vi "ComplexWaveformVisualizer.vi"(6 "new?":bool=TRUE, 8 "imag":dbl[](array[numeric]), 9 "real":dbl[](array[numeric]), 10 "dt":dbl format="%#_13g", 11 "t0":dbl format="%#_13g") -> (0 "error out":errorcluster)   [LabVIEW 2018, in "lvnetviz.lvlib" / "ComplexWaveform.lvclass"]
uses:
  ComplexWaveform.lvclass
  37a200e1-ebed-4a42-aca9-62fa0edddda8.vi
  563f4c1e-5713-48a9-8981-6f50fa41d22c.vi
  e92ec0bc-6cb3-4747-b161-0f80a961e92f.vi
  60cc32db-fe2c-4d93-b9a7-8d3187e357da.vi
  692aab13-ca21-4d55-90b4-8dcecc026462.vi
  02b4f178-3a94-4fae-b2df-360b2a148257.vi
  3b6274d3-9685-4d49-9d46-acf0fd8be449.vi
  563f4c1e-5713-48a9-8981-6f50fa41d22c.vi/40b995cc-7a2b-45c3-8b81-c77e08a5a566.vi
  e92ec0bc-6cb3-4747-b161-0f80a961e92f.vi/273ea279-4d78-4cbc-b357-74e972452477.vi
  <vilib>/Analysis/2dsp.llb/Unwrap Phase.vi
  <vilib>/Analysis/2dsp.llb/FFT.vi
  <vilib>/Analysis/2dsp.llb/Complex FFT.vi
  e92ec0bc-6cb3-4747-b161-0f80a961e92f.vi/273ea279-4d78-4cbc-b357-74e972452477.vi/7830e0d0-7296-4e8f-a228-935442eb8294.vi
  <vilib>/Utility/error.llb/Error Cluster From Error Code.vi
panel:
  in  "Tab Control":enum32{"Traces", "Statistics"}(tab)
  out "Waveform Graph":cluster{"t0":dbl, "dt":dbl, "real":dbl[]}[](graph)
  in  "Plot Type":T1(ring)=enum."Power vs. Frequency"
  out "Table Control":string[][](table)
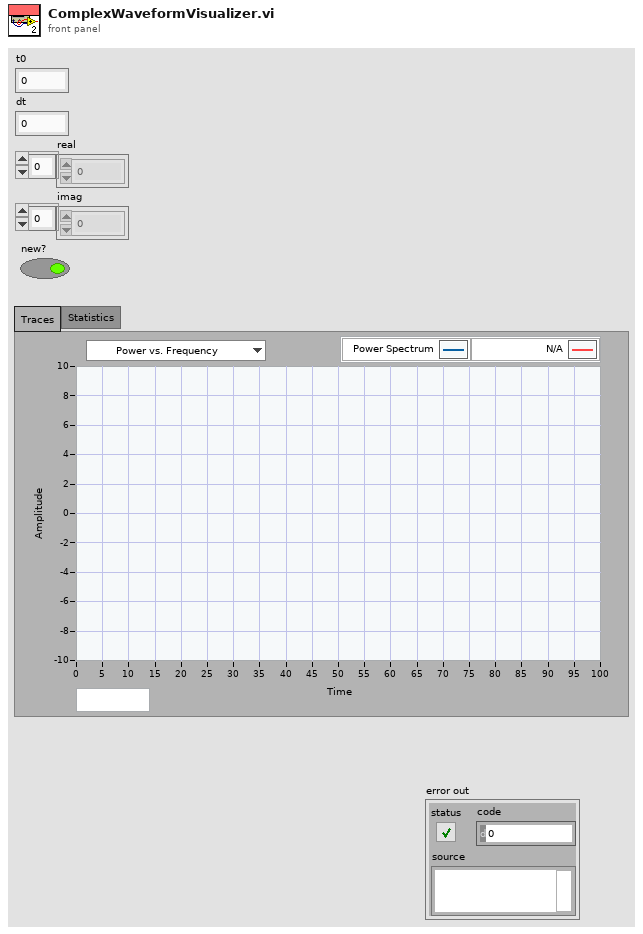
[diagram p1: front panel]
types:
  T1 = enum16{"IQ vs. Time", "Power vs. Time", "Phase vs. Time", "Unwrapped Phase vs. Time", "Delta Phase vs. Time", "Frequency vs. Time", "Power vs. Frequency", "Phase vs. Frequency"}
  T2 = cluster{"t0":dbl, "dt":dbl, "Unwrapped Phase":dbl[]}
  T3 = cluster{"t0":dbl, "dt":dbl, "Unwrapped Phase":dbl[]}[]
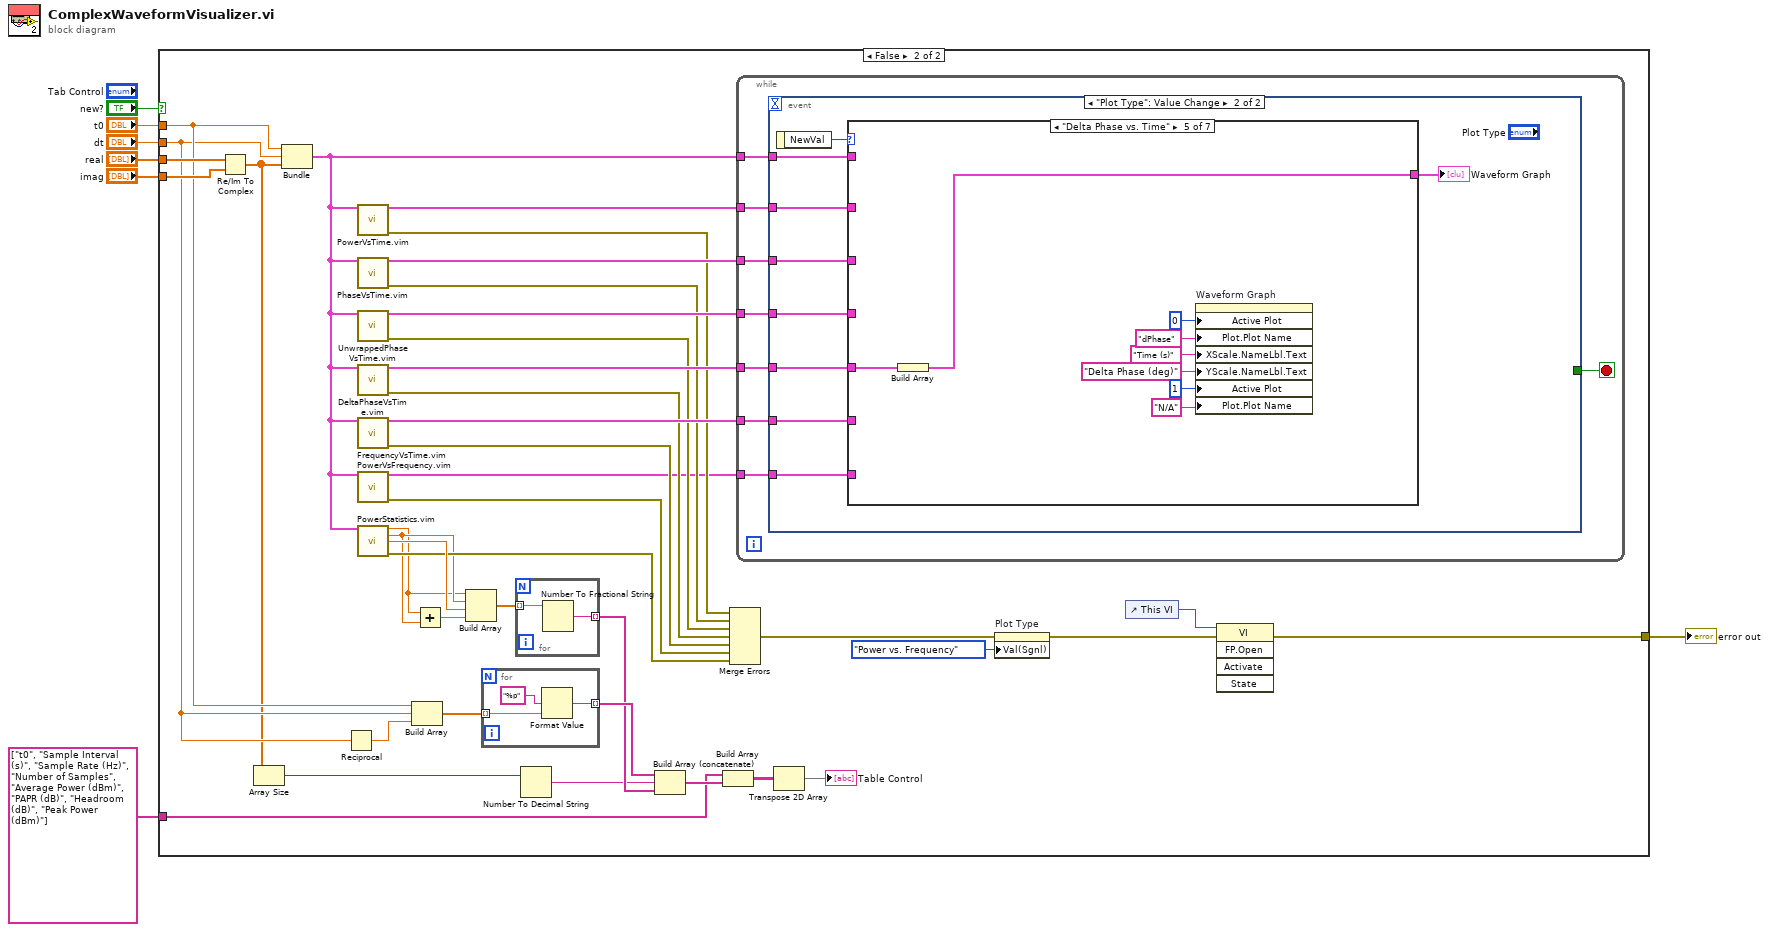
[diagram p0: block diagram]
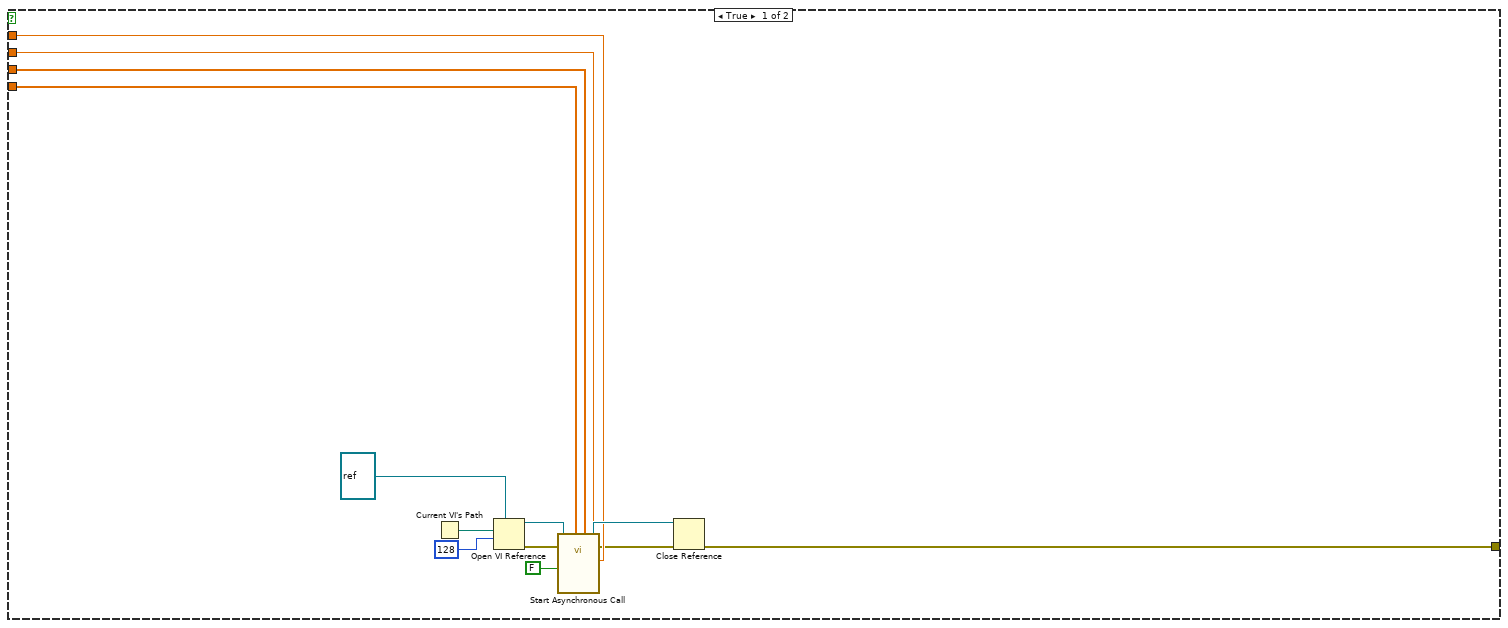
[diagram p2: hidden frame]
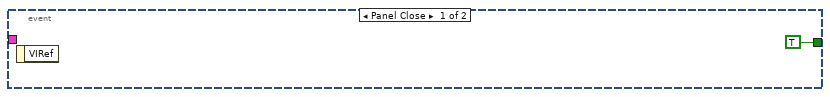
[diagram p3: hidden frame]
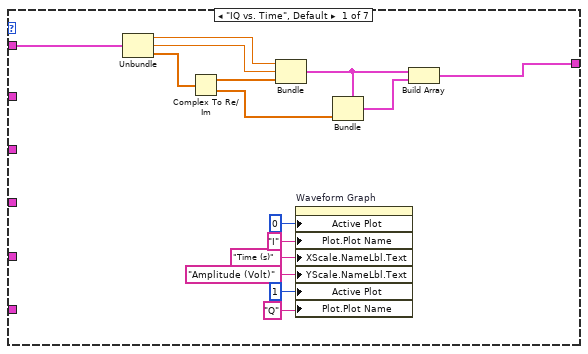
[diagram p4: hidden frame]
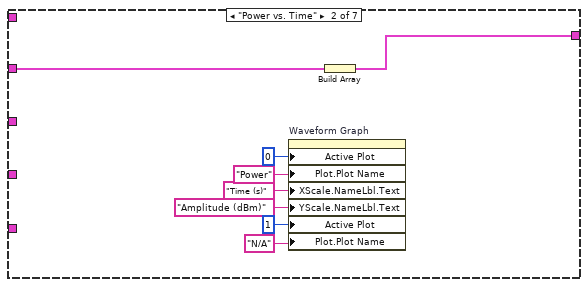
[diagram p5: hidden frame]
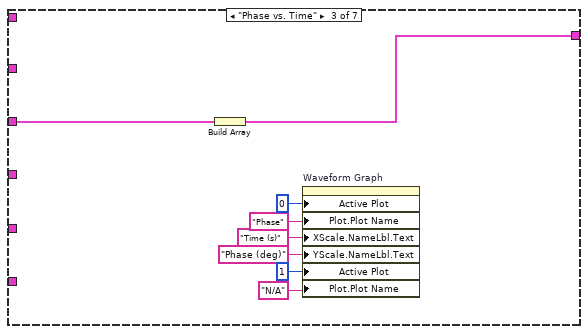
[diagram p6: hidden frame]
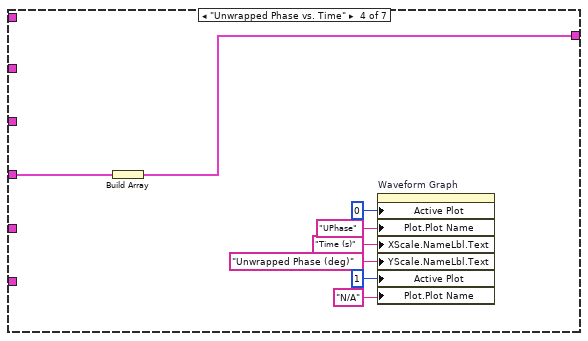
[diagram p7: hidden frame]
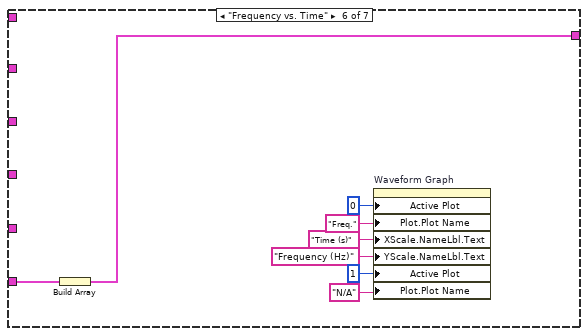
[diagram p8: hidden frame]
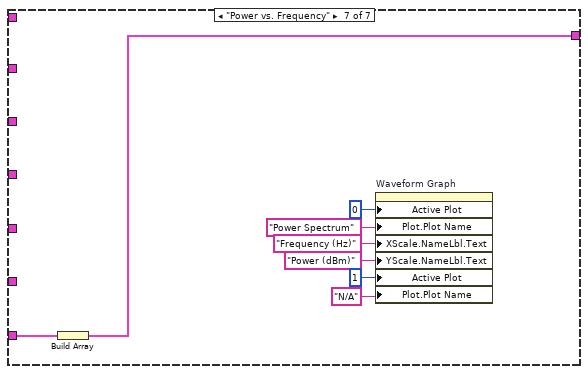
[diagram p9: hidden frame]
diagram:
  n1 = case shown="False" "new?" {
    tunnel: "imag" -> [w12 w52]
    tunnel: "real" -> [w13 w53]
    tunnel: "t0" -> [w15 w48]
    tunnel: "dt" -> [w14 w41]
    tunnel: [w9 w58] -> w2
    tunnel: string[] ["t0", "Sample Interval (s)", "Sample Rate (Hz)", "Number of Samples", "Average Power (dBm)", "PAPR (dB)", "Headroom (dB)", "Peak Power (dBm)"] -> [_ w35]
    frame True {
      n2 = Current VI's Path() -> (path=w20:path)
      n3 = Open VI Reference(type specifier VI Refnum (for type only)=refnum<vi> refnum, vi path=w20, options=128) -> (vi reference=w17:refnum<vi>, error out=w11:errorcluster)  [unwired: 3 in]
      n4 = call-by-ref "Start Asynchronous Call"(reference=w17, error in=w11, "Create New?"=FALSE, "imag"=w12, "real"=w13, "dt"=w14, "t0"=w15) -> (reference out=w16:refnum<vi>, error out=w10:errorcluster)  [unwired: 6 in, 1 out]
      n5 = Close Reference(reference=w16, error in (no error)=w10) -> (error out=w9:errorcluster)
    }
    frame False {
      n6 = Re/Im To Complex(1:w52, 2:w53) -> (0:w39:cdb[])
      n7 = Array Size(array=w39) -> (size(s)=w38:i32)
      n8 = Bundle("t0"=w48, "dt"=w41, w39) -> (w42:cluster{"t0":dbl, "dt":dbl, cdb[]})  [unwired: 1 in]
      n9 = Reciprocal(x=w41) -> (1/x=w40:dbl)
      n10 = call "PowerVsTime.vim"("Complex Waveform"=w42) -> ("Power vs. Time"=w47:cluster{"t0":dbl, "dt":dbl, dbl[]}, "error out"=w34:errorcluster)  [unwired: 13 in]
      n11 = call "PhaseVsTime.vim"("Complex Waveform"=w42) -> ("Phase vs. Time (deg)"=w46:cluster{"t0":dbl, "dt":dbl, dbl[]}, "error out"=w33:errorcluster)  [unwired: 13 in]
      n12 = call "UnwrappedPhaseVsTime.vim"("Complex Waveform"=w42) -> ("Unwrapped Phase vs. Time (deg)"=w45:T2, "error out"=w32:errorcluster)  [unwired: 13 in]
      n13 = call "DeltaPhaseVsTime.vim"("Complex Waveform"=w42) -> ("Delta Phase vs. Time (deg)"=w44:cluster{dbl, "dt":dbl, dbl[]}, "error out"=w31:errorcluster)  [unwired: 13 in]
      n14 = call "FrequencyVsTime.vim"("Complex Waveform"=w42) -> ("Frequency vs. Time (Hz)"=w43:cluster{dbl, "dt":dbl, dbl[]}, "error out"=w30:errorcluster)  [unwired: 13 in]
      n15 = call "PowerVsFrequency.vim"("Complex Waveform"=w42) -> ("Power vs. Frequency"=w27:cluster{dbl, dbl, dbl[]}, "error out"=w29:errorcluster)  [unwired: 13 in]
      n16 = call "PowerStatistics.vim"("Complex Waveform"=w42) -> ("Average Power (dBm)"=w22:dbl, "PAPR (dB)"=w23:dbl, "Headroom (dB)"=w57:dbl, "error out"=w28:errorcluster)  [unwired: 11 in]
      n17 = Build Array(w48, w41, w40) -> (w49:dbl[])
      n18 = Add(x=w22, y=w23) -> (x+y=w21:dbl)
      n19 = Build Array(w22, w23, w57, w21) -> (w56:dbl[])
      n20 = for {
        tunnel: [w61] -> w50 mode=indexing
        tunnel: w49 -> [w60] mode=indexing
        n21 = Format Value(format string="%p", value (0)=w60) -> (output string=w61:string)  [unwired: 1 in]
      }
      n22 = for {
        tunnel: [w64] -> w37 mode=indexing
        tunnel: w56 -> [w63] mode=indexing
        n23 = Number To Fractional String(number=w63) -> (F-format string=w64:string)  [unwired: 3 in]
      }
      n24 = Number To Decimal String(number=w38) -> (decimal integer string=w36:string)  [unwired: 1 in]
      n25 = Build Array (concatenate)(w50, w36, w37) -> (w51:string[])
      n26 = Build Array(w35, w51) -> (w55:string[][])
      n27 = Merge Errors(w34, w33, w32, w31, w30, w29, w28) -> (w26:errorcluster)
      n28 = while {
        tunnel: w42 -> [w71]
        tunnel: w47 -> [w70]
        tunnel: w46 -> [w69]
        tunnel: w45 -> [w68]
        tunnel: w44 -> [w67]
        tunnel: w43 -> [w66]
        tunnel: w27 -> [w65]
        stop <- w72 stop-if-true
        n29 = event shown="[1] \"Plot Type\": Value Change" {
          selector: _ -> [_ _]
          dyn-events: _ -> [_ _]
          timeout: _ -> [_ _]
          tunnel: [TRUE _] -> w72
          tunnel: w71 -> [_ w81]
          tunnel: w70 -> [_ w80]
          tunnel: w69 -> [_ w79]
          tunnel: w68 -> [_ w78]
          tunnel: w67 -> [_ w77]
          tunnel: w66 -> [_ w76]
          tunnel: w65 -> [_ w75]
          event Panel Close {
            n30 = event-data() -> ()  [unwired: 1 in, 1 out]
          }
          event "Plot Type": Value Change {
            n31 = event-data() -> ("NewVal"=w82:T1)  [unwired: 1 in]
            n32 = case shown="\"Delta Phase vs. Time\"" w82 {
              tunnel: [w89 w105 w112 w120 w122 w130 w138] -> w74
              tunnel: w81 -> [w97 _ _ _ _ _ _]
              tunnel: w80 -> [_ w104 _ _ _ _ _]
              tunnel: w79 -> [_ _ w113 _ _ _ _]
              tunnel: w78 -> [_ _ _ w121 _ _ _]
              tunnel: w77 -> [_ _ _ _ w123 _ _]
              tunnel: w76 -> [_ _ _ _ _ w131 _]
              tunnel: w75 -> [_ _ _ _ _ _ w139]
              frame "IQ vs. Time", Default {
                n33 = Unbundle(w97) -> ("t0"=w94:dbl, "dt"=w93:dbl, w96:cdb[])
                n34 = Complex To Re/Im(x + iy=w96) -> (x=w95:dbl[], y=w92:dbl[])
                n35 = Bundle("t0"=w94, "dt"=w93, w95) -> (w91:cluster{"t0":dbl, "dt":dbl, dbl[]})  [unwired: 1 in]
                n36 = property on="Waveform Graph" class="WFGraph (strict)"("Active Plot"=u32 0, "Plot.Plot Name"="I", "XScale.NameLbl.Text"="Time (s)" ("X Scale.Name Label.Text"), "YScale.NameLbl.Text"="Amplitude (Volt)" ("Y Scale.Name Label.Text"), "Active Plot"=u32 1, "Plot.Plot Name"="Q") -> ()  [unwired: 2 in, 2 out]
                n37 = Bundle(cluster=w91, w92) -> (w90:cluster{"t0":dbl, "dt":dbl, dbl[]})  [unwired: 2 in]
                n38 = Build Array(w91, w90) -> (w89:cluster{"t0":dbl, "dt":dbl, dbl[]}[])
              }
              frame "Power vs. Time" {
                n39 = property on="Waveform Graph" class="WFGraph (strict)"("Active Plot"=u32 0, "Plot.Plot Name"="Power", "XScale.NameLbl.Text"="Time (s)" ("X Scale.Name Label.Text"), "YScale.NameLbl.Text"="Amplitude (dBm)" ("Y Scale.Name Label.Text"), "Active Plot"=u32 1, "Plot.Plot Name"="N/A") -> ()  [unwired: 2 in, 2 out]
                n40 = Build Array(w104) -> (w105:cluster{"t0":dbl, "dt":dbl, dbl[]}[])
              }
              frame "Phase vs. Time" {
                n41 = Build Array(w113) -> (w112:cluster{"t0":dbl, "dt":dbl, dbl[]}[])
                n42 = property on="Waveform Graph" class="WFGraph (strict)"("Active Plot"=u32 0, "Plot.Plot Name"="Phase", "XScale.NameLbl.Text"="Time (s)" ("X Scale.Name Label.Text"), "YScale.NameLbl.Text"="Phase (deg)" ("Y Scale.Name Label.Text"), "Active Plot"=u32 1, "Plot.Plot Name"="N/A") -> ()  [unwired: 2 in, 2 out]
              }
              frame "Unwrapped Phase vs. Time" {
                n43 = Build Array(w121) -> (w120:T3)
                n44 = property on="Waveform Graph" class="WFGraph (strict)"("Active Plot"=u32 0, "Plot.Plot Name"="UPhase", "XScale.NameLbl.Text"="Time (s)" ("X Scale.Name Label.Text"), "YScale.NameLbl.Text"="Unwrapped Phase (deg)" ("Y Scale.Name Label.Text"), "Active Plot"=u32 1, "Plot.Plot Name"="N/A") -> ()  [unwired: 2 in, 2 out]
              }
              frame "Delta Phase vs. Time" {
                n45 = Build Array(w123) -> (w122:cluster{dbl, "dt":dbl, dbl[]}[])
                n46 = property on="Waveform Graph" class="WFGraph (strict)"("Active Plot"=u32 0, "Plot.Plot Name"="dPhase", "XScale.NameLbl.Text"="Time (s)" ("X Scale.Name Label.Text"), "YScale.NameLbl.Text"="Delta Phase (deg)" ("Y Scale.Name Label.Text"), "Active Plot"=u32 1, "Plot.Plot Name"="N/A") -> ()  [unwired: 2 in, 2 out]
              }
              frame "Frequency vs. Time" {
                n47 = Build Array(w131) -> (w130:cluster{dbl, "dt":dbl, dbl[]}[])
                n48 = property on="Waveform Graph" class="WFGraph (strict)"("Active Plot"=u32 0, "Plot.Plot Name"="Freq.", "XScale.NameLbl.Text"="Time (s)" ("X Scale.Name Label.Text"), "YScale.NameLbl.Text"="Frequency (Hz)" ("Y Scale.Name Label.Text"), "Active Plot"=u32 1, "Plot.Plot Name"="N/A") -> ()  [unwired: 2 in, 2 out]
              }
              frame "Power vs. Frequency" {
                n49 = Build Array(w139) -> (w138:cluster{dbl, dbl, dbl[]}[])
                n50 = property on="Waveform Graph" class="WFGraph (strict)"("Active Plot"=u32 0, "Plot.Plot Name"="Power Spectrum", "XScale.NameLbl.Text"="Frequency (Hz)" ("X Scale.Name Label.Text"), "YScale.NameLbl.Text"="Power (dBm)" ("Y Scale.Name Label.Text"), "Active Plot"=u32 1, "Plot.Plot Name"="N/A") -> ()  [unwired: 2 in, 2 out]
              }
            }
            "Waveform Graph" <- w74
          }
        }
      }
      n51 = Transpose 2D Array(2D array=w55) -> (transposed array=→"Table Control":string[][])
      n52 = property on="Plot Type" class="Enum (strict)"(error in=w26, "Val(Sgnl)"=T1."Power vs. Frequency" ("Value (Signaling)")) -> (error out=w25:errorcluster)  [unwired: 1 in, 1 out]
      n53 = control-ref of="This VI"() -> (w59:refnum<vi>)
      n54 = invoke class="VI" method="FP.Open"(reference=w59, error in=w25) -> (error out=w58:errorcluster)  [unwired: 3 in, 4 out]
    }
  }
  "error out" <- w2
